vi "Generate UI Mesage UE.vi"(8 "error in (no error)":errorcluster, 10 "UI Message":string, 11 "Project Sync Tools in":refnum<class "Project Sync Tools.lvclass">) -> (0 "error out":errorcluster, 3 "Project Sync Tools out":refnum<class "Project Sync Tools.lvclass">)   [LabVIEW 2019, in "Project Sync Tools.lvclass"]
uses:
  Project Sync Tools.lvclass
  Project Sync Tools.lvclass/Project Sync Tools.ctl
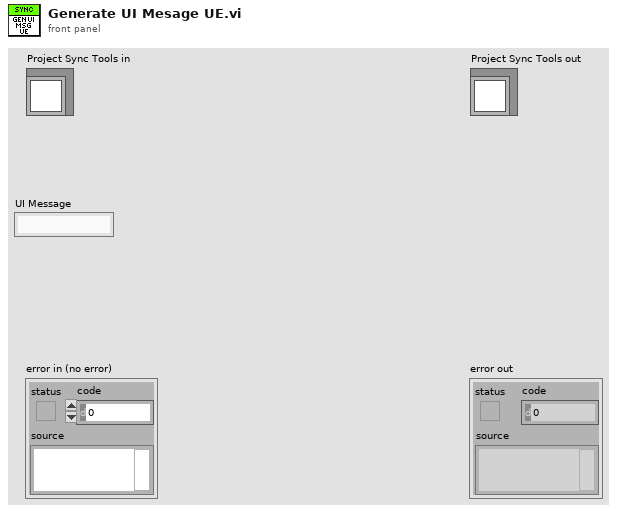
[diagram p1: front panel]
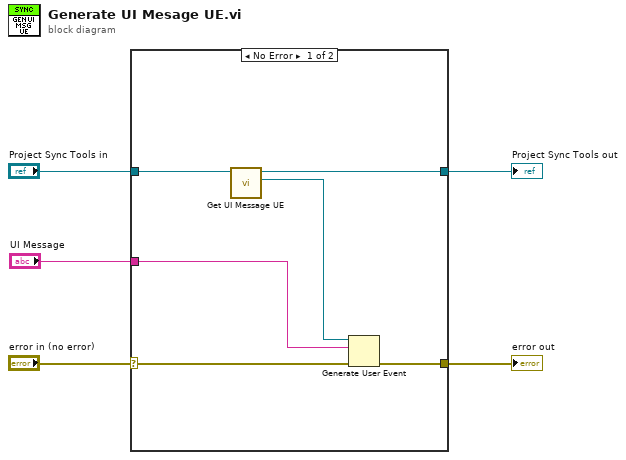
[diagram p0: block diagram]
diagram:
  n1 = case shown="No Error" "error in (no error)" {
    selector: "error in (no error)" -> [w9 w13]
    tunnel: [w8 w13] -> w4
    tunnel: [w7 w12] -> w2
    tunnel: "Project Sync Tools in" -> [w11 w12]
    tunnel: "UI Message" -> [w6 _]
    frame No Error {
      n2 = call "Get UI Message UE.vi"("Project Sync Tools in"=w11) -> ("UI Message UE"=w10:refnum<user-event>, "Project Sync Tools out"=w7:refnum<class "Project Sync Tools.lvclass">)  [unwired: 9 in]
      n3 = Generate User Event(user event=w10, event data cluster=w6, error in=w9) -> (error out=w8:errorcluster)  [unwired: 1 in, 1 out]
    }
    frame Error {
    }
  }
  "error out" <- w4
  "Project Sync Tools out" <- w2
